vi "retrieve-can-data.vi"(8 "error in (no error)":errorcluster, 9 "id":u32 format="%.0x", 11 "CANtable in":refnum<class "bAPPdata.lvclass">) -> (0 "error out":errorcluster, 1 "CAN frame":T1 {"payload" format="%x"; "timestamp" format="%<%.7X\n%x>T"; "type" items=["CAN Data"=0, "CAN Remote"=1, "CAN Bus Error"=2, "J1939 Data"=192, "Delay"=224, "Log Trigger"=225, "Start Trigger"=226]; "identifier" format="%x"}, 3 "CANtable out":refnum<class "bAPPdata.lvclass">)   [LabVIEW 2015, in "bAPPdata.lvclass"]
uses:
  bAPPdata.lvclass
  <vilib>/xnet/xnet.llb/XNET Frame CAN.ctl
  <vilib>/xnet/xnet.llb/XNET Frame Type CAN.ctl
  bAPPdata.lvclass/bAPPdata.ctl
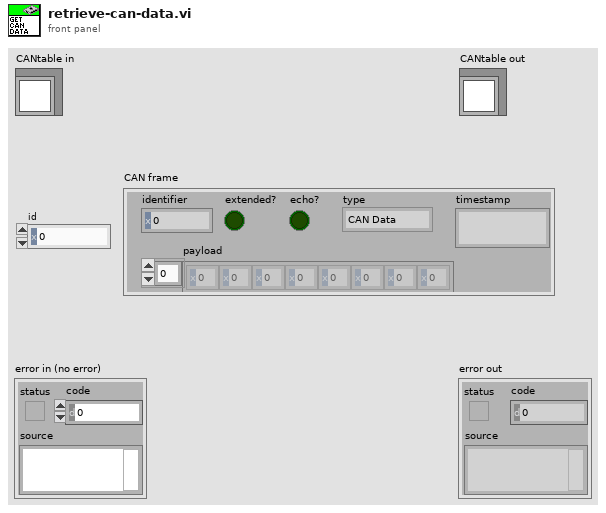
[diagram p1: front panel]
types:
  T1 = typedef "XNET Frame CAN.ctl" = cluster{"timestamp":timestamp, "payload":u8[], "identifier":u32, "type":T2, "extended?":bool, "echo?":bool}
  T2 = typedef "XNET Frame Type CAN.ctl" = u8
  T3 = typedef "bAPPdata.lvclass/table-data.ctl" = T4[]
  T4 = typedef "bAPPdata.lvclass/table-contents.ctl" = cluster{"id":u32, "tag":string, "frame.type":T5, "last.frame":T1, "tMsgData":T6, "child.tags":string[], "bit-payload":bool[]}
  T5 = typedef "frame.type.ctl" = enum16{"FRAME NOT DEFINED", "DUT OUTPUT FRAME", "DUT INPUT FRAME"}
  T6 = typedef "nMsgData.ctl" = cluster{"dwID":u32, "count":u32, "dwCycleTime":dbl, "dwTime":dbl, "new msg":bool}
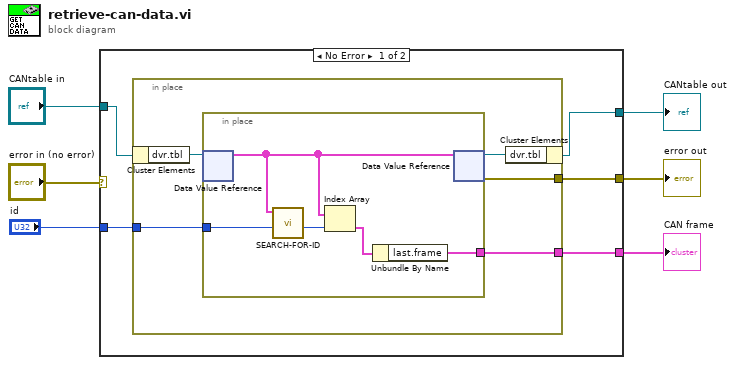
[diagram p0: block diagram]
diagram:
  n1 = case shown="No Error" "error in (no error)" {
    selector: "error in (no error)" -> [_ w23]
    tunnel: [w7 w23] -> w5
    tunnel: [w10 w22] -> w3
    tunnel: "CANtable in" -> [w11 w22]
    tunnel: "id" -> [w9 _]
    tunnel: [w8 _] -> w1
    frame No Error {
      n2 = in-place {
        in-place-border: [w14] -> w7
        in-place-border: w9 -> [w13]
        in-place-border: [w12] -> w8
        n3 = in-place-cluster #1(w11) -> ("dvr.tbl"=w16:refnum<data-value>)
        n4 = in-place {
          in-place-border: w13 -> [w21]
          in-place-border: [w20] -> w12
          n5 = in-place-dvr #2(w16) -> (w17:T3)  [unwired: 1 out]
          n6 = call "SEARCH-FOR-ID.vi"("ID"=w21, "tbl.list"=w17) -> ("idx"=w18:i32)  [unwired: 8 in, 1 out]
          n7 = Index Array(array=w17, index=w18) -> (element=w19:T4)
          n8 = Unbundle By Name(w19) -> ("last.frame"=w20:T1)
          n9 = in-place-dvr #2(w17) -> (w15:refnum<data-value>, w14:errorcluster)
        }
        n10 = in-place-cluster #1("dvr.tbl"=w15) -> (w10:refnum<class "bAPPdata.lvclass">)
      }
    }
    frame Error {
    }
  }
  "error out" <- w5
  "CANtable out" <- w3
  "CAN frame" <- w1
